vi "processing_steps.vi"(1 "input cluster":T3) -> (0 "output cluster":T1)   [LabVIEW 2010]
uses:
  <vilib>/vision/Image Controls.llb/IMAQ Image.ctl
  lib/MWT.dll
  <vilib>/vision/NI_Vision_Development_Module.lvlib
panel:
  out "Image Pixels (I16) 3":i16[][](array[numeric])
  out "Image Pixels (I16) 2":i16[][](array[numeric])
  out "element 2":i32
  out "element":i32
  out "return type":i32
  out "error out":errorcluster
  out "Numeric":i32
  out "Image Out":T2
  out "Image Pixels (I16)":i16[][](array[numeric])
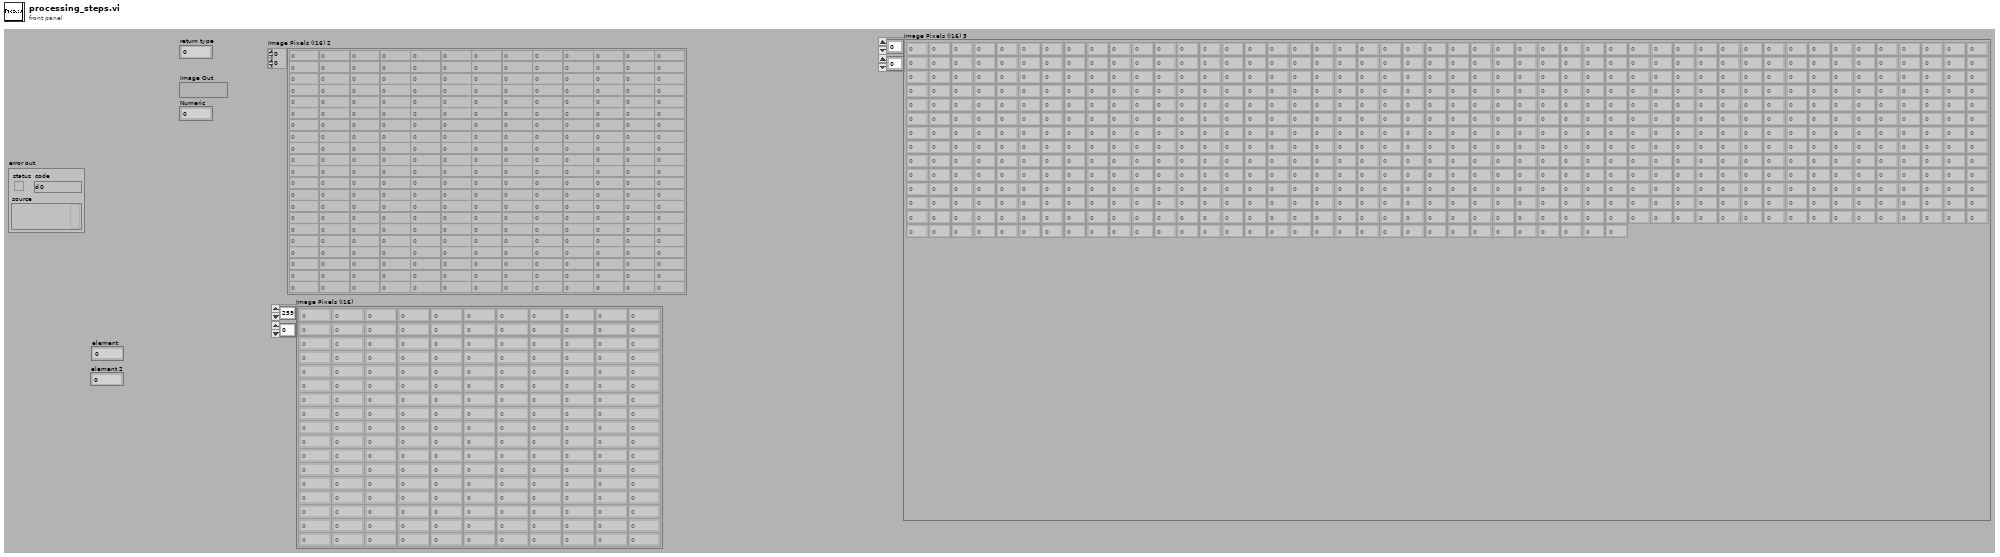
[diagram p1: front panel]
types:
  T1 = cluster{"return value":i32, "return value":i32, "Image Pixels (I16) out":i16[][], "coordinates":i32[]}
  T2 = typedef "IMAQ Image.ctl" = refnum<image>
  T3 = cluster{i32, "Value":i32, "Value":u16, sgl, "Value":u16, "Value":bool, "Value":u32, "Image Out":T2, "Image Pixels (I16)":i16[][], i32[]}
  T4 = typedef "Image Type" = u32
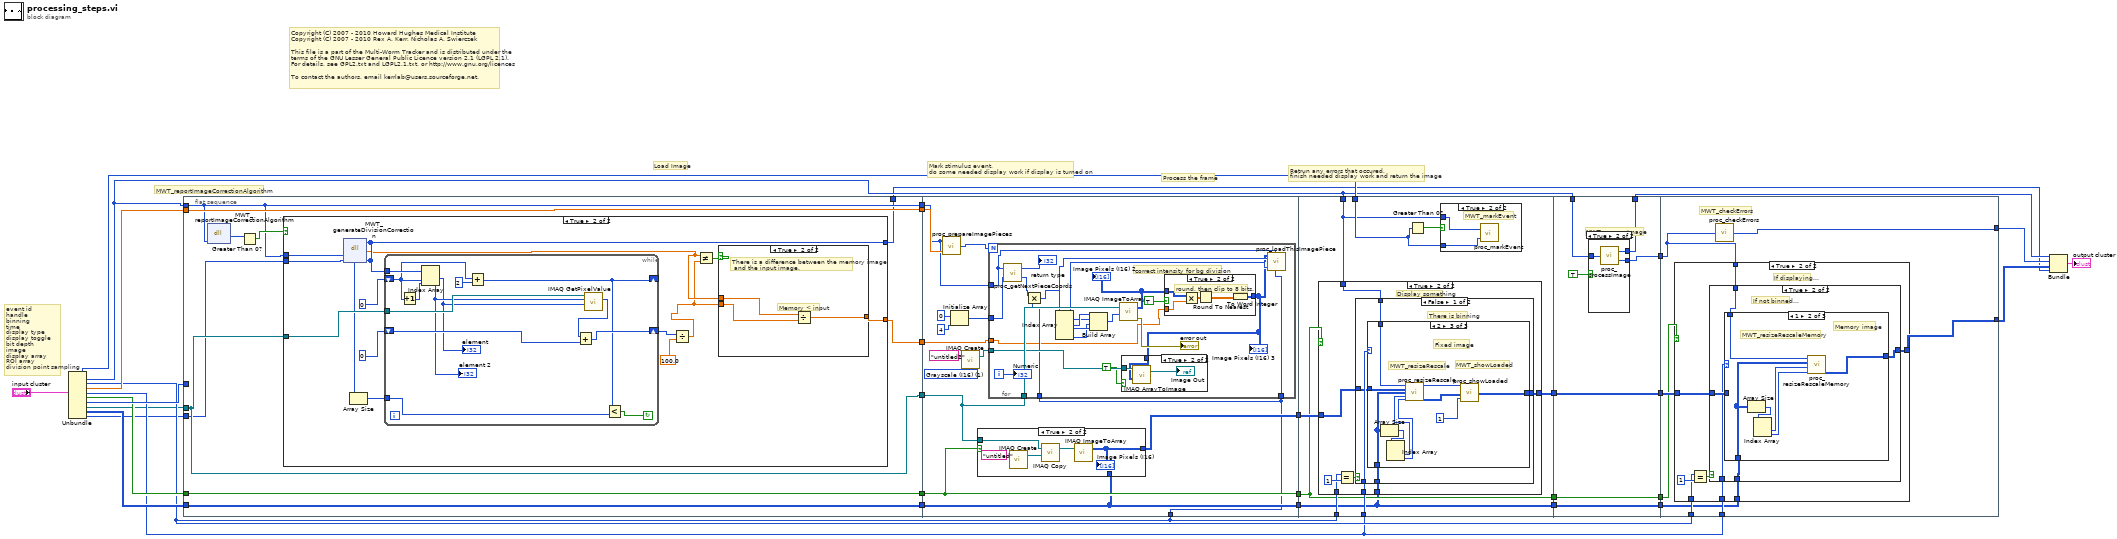
[diagram p0: block diagram]
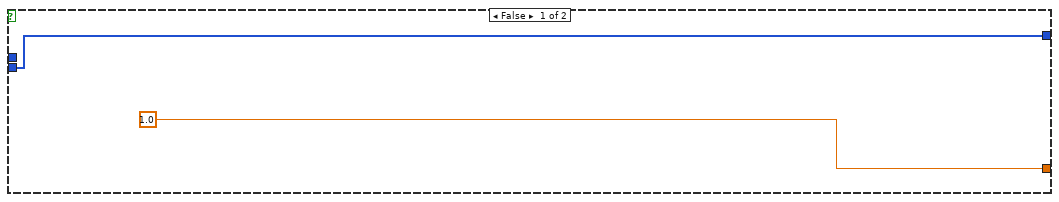
[diagram p2: hidden frame]
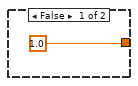
[diagram p3: hidden frame]
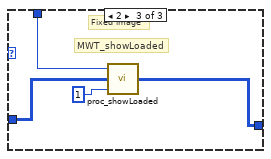
[diagram p12: hidden frame]
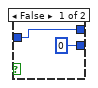
[diagram p14: hidden frame]
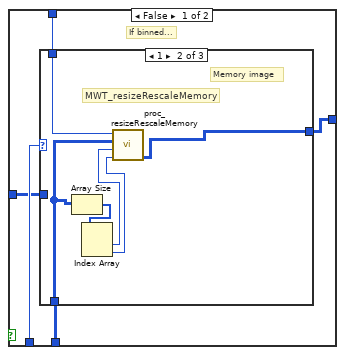
[diagram p16: hidden frame]
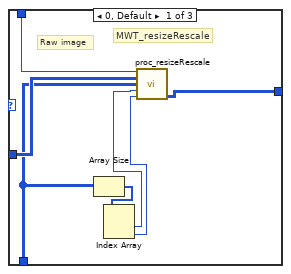
[diagram p17: hidden frame]
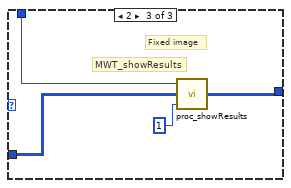
[diagram p18: hidden frame]
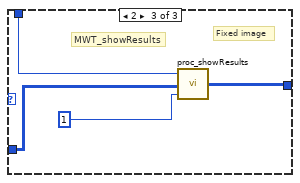
[diagram p20: hidden frame]
diagram:
  # "MWT_reportImageCorrectionAlgorithm"
  # "Copyright (C) 2007 - 2010 Howard Hughes Medical Institute\nCopyright (C) 2007 - 2010 Rex A. Kerr, Nicholas A. Swierczek\n \nThis file is a part of the Multi-Worm Tracker and is distributed under the\nterms of the GNU Lesser General Public Licence version 2.1 (LGPL 2.1).\nFor details, see GPL2.txt and LGPL2.1.txt, or http://www.gnu.org/licences\n \nTo contact the authors, email kerrlab@users.sourceforge.net."
  # "Retrun any errors that occured,\nfinish needed display work and return the image"
  # "Process the frame"
  # "Mark stimulus event,\ndo some needed display work if display is turned on"
  # "Load Image"
  # "event id\nhandle\nbinning\ntime\ndisplay type\ndisplay toggle\nbit depth\nimage\ndisplay array\nROI array\ndivision point sampling"
  n1 = Unbundle("input cluster") -> (w30:i32, "Value"=w5:i32, "Value"=w24:u16, w31:sgl, "Value"=w23:u16, "Value"=w26:bool, "Value"=w32:u32, "Image Out"=w12:T2, "Image Pixels (I16)"=w25:i16[][], w3:i32[])
  n2 = flat-sequence {
    tunnel: w25 -> [w40]
    tunnel: w26 -> [w41]
    tunnel: w5 -> [w36]
    tunnel: w32 -> [_]
    tunnel: w12 -> [w39]
    tunnel: w31 -> [w42]
    tunnel: [w42] -> w11
    tunnel: [w39] -> w10
    tunnel: [w36] -> w9
    tunnel: [w41] -> w8
    tunnel: [w40] -> w7
    tunnel: [w35] -> w6
    tunnel: w3 -> [w34]
    tunnel: [w33] -> w2
    tunnel: [w88] -> w22
    tunnel: [w89] -> w21
    tunnel: [w87] -> w20
    tunnel: w24 -> [w76]
    tunnel: w11 -> [w79]
    tunnel: w10 -> [w83]
    tunnel: w9 -> [w77]
    tunnel: w8 -> [w89]
    tunnel: w7 -> [w87]
    tunnel: w6 -> [w75]
    tunnel: w30 -> [w133]
    tunnel: w24 -> [w132]
    tunnel: w5 -> [w131]
    tunnel: w23 -> [w130]
    tunnel: [w129] -> w19
    tunnel: w22 -> [w128]
    tunnel: w21 -> [w127]
    tunnel: [w127] -> w18
    tunnel: w20 -> [w126]
    tunnel: [w126] -> w17
    tunnel: [w179] -> w16
    tunnel: [w180] -> w27
    tunnel: w5 -> [w178]
    tunnel: [w177] -> w15
    tunnel: w19 -> [w177]
    tunnel: [w176] -> w14
    tunnel: w18 -> [w176]
    tunnel: [w175] -> w13
    tunnel: w17 -> [w175]
    tunnel: w16 -> [w191]
    tunnel: [w190] -> w28
    tunnel: [w193] -> w29
    tunnel: w24 -> [w192]
    tunnel: w23 -> [w189]
    tunnel: w15 -> [w188]
    tunnel: w14 -> [w187]
    tunnel: w13 -> [w186]
    frame #0 {
      n3 = dll-call lib="C:/MWT/lib/MWT.dll" fn="MWT_reportImageCorrectionAlgorithm"("handle"=w36) -> ("return type"=w38:i32)  [unwired: 4 in, 2 out]
      n4 = Greater Than 0?(x=w38) -> (x > 0?=w37:bool)
      n5 = case shown="True" w37 {
        tunnel: w36 -> [_ w57]
        tunnel: w39 -> [_ w54]
        tunnel: [1.0 w52] -> w35
        tunnel: w34 -> [w43 w49]
        tunnel: [w43 w48] -> w33
        frame False {
        }
        frame True {
          n6 = dll-call lib="C:/MWT/lib/MWT.dll" fn="MWT_generateDivisionCorrection"("handle"=w57, "coordinates"=w49) -> ("return type"=w47:sgl, "coordinates"=w48:i32[])  [unwired: 4 in, 2 out]
          n7 = Array Size(array=w48) -> (size(s)=w45:i32)
          n8 = while {
            shift-right: [w59] -> _
            shift-left: 0 -> [w67]
            tunnel: w48 -> [w69]
            tunnel: w54 -> [w66]
            shift-right: [w63] -> w50
            shift-left: i16 0 -> [w64]
            tunnel: w45 -> [w58]
            stop <- w60 continue-if-true
            n9 = Increment(x=w67) -> (x+1=w70:i32)
            n10 = Index Array(array=w69, index #1=w67, index #2=w70) -> (element #1=w61:i32, element #2=w62:i32)
            "element" <- w61
            "element 2" <- w62
            n11 = Add(x=w67, y=2) -> (x+y=w59:i32)
            n12 = call "IMAQ GetPixelValue"("Image"=w66, "X Coordinate"=w62, "Y Coordinate"=w61) -> ("Pixel Value (I16)"=w65:i16)  [unwired: 3 in, 4 out]
            n13 = Add(x=w65, y=w64) -> (x+y=w63:i16)
            n14 = Less?(x=w59, y=w58) -> (x < y?=w60:bool)
          }
          n15 = Divide(x=w50, y=sgl 100.0) -> (x/y=w46:sgl)
          n16 = Not Equal?(x=w47, y=w46) -> (x != y?=w53:bool)
          n17 = case shown="True" w53 {
            tunnel: w47 -> [_ w74]
            tunnel: w46 -> [_ w73]
            tunnel: [1.0 w72] -> w52
            frame False {
            }
            frame True {
              # "Memory < input"
              # "There is a difference between the memory image\n and the input image."
              n18 = Divide(x=w74, y=w73) -> (x/y=w72:sgl)
            }
          }
        }
      }
    }
    frame #1 {
      w80 = T4 1 items=["Grayscale (U8)", "Grayscale (I16)", "Grayscale (SGL)", "Complex (CSG)", "RGB (U32)", "HSL (U32)", "RGB (U64)"] ("Image Type")
      n19 = call "proc_prepareImagePieces.vi"("time"=w79, "handle"=w77) -> ("piece count"=w78:i32)
      n20 = Initialize Array(0 ("element"), 4 ("dimension size")) -> (w84:i32[])
      n21 = call "IMAQ Create"("Image Name"="untitled2", "Image Type"=w80) -> ("New Image"=w81:T2)  [unwired: 3 in, 1 out]
      n22 = case shown="True" w89 {
        tunnel: [w120 w125] -> w88
        tunnel: w87 -> [w120 _]
        tunnel: w83 -> [_ w121]
        frame False {
        }
        frame True {
          n23 = call "IMAQ Create"("Image Name"="untitled") -> ("New Image"=w123:T2)  [unwired: 4 in, 1 out]
          n24 = call "IMAQ Copy"("Image Dst"=w123, "Image Src"=w121) -> ("Image Dst Out"=w122:T2)  [unwired: 4 in, 1 out]
          n25 = call "IMAQ ImageToArray"("Image"=w122) -> ("Image Pixels (I16)"=w125:i16[][])  [unwired: 3 in, 4 out]
          "Image Pixels (I16)" <- w125
        }
      }
      n26 = for {
        N: w78 -> [_]
        tunnel: w77 -> [w104]
        tunnel: w84 -> [w106]
        tunnel: w83 -> [w110]
        tunnel: w81 -> [w109]
        tunnel: w76 -> [w97]
        tunnel: w76 -> [w96]
        tunnel: w75 -> [w90]
        i -> [w108]
        # "correct intensity for bg division"
        n27 = call "proc_getNextPieceCoords.vi"("initialized array"=w106, "handle"=w104) -> ("coordinates"=w95:i32[], "returned handle"=→"return type":i32)
        n28 = Multiply(x=w95, y=w96) -> (x*y=w94:i32[])
        n29 = Index Array(array=w94) -> (element #1=w99:i32, element #2=w100:i32, element #3=w103:i32, element #4=w102:i32)  [unwired: 4 in]
        n30 = Build Array(w100, w99, w102, w103) -> (w98:i32[])
        n31 = call "IMAQ ImageToArray"("Optional Rectangle"=w98, "Image"=w110) -> ("error out"=→"error out":errorcluster, "Image Pixels (I16)"=w92:i16[][])  [unwired: 2 in, 3 out]
        "Image Pixels (I16) 2" <- w92
        n32 = case shown="True" TRUE {
          tunnel: w90 -> [_ w116]
          tunnel: [w111 w113] -> w93
          tunnel: w92 -> [w111 w115]
          frame False {
          }
          frame True {
            # "round, then clip to 8 bits."
            n33 = Multiply(x=w115, y=w116) -> (x*y=w114:dbl[][])
            n34 = Round To Nearest(number=w114) -> (nearest integer value=w112:dbl[][])
            n35 = To Word Integer(number=w112) -> (16bit integer=w113:i16[][])
          }
        }
        "Image Pixels (I16) 3" <- w93
        n36 = case shown="True" TRUE {
          tunnel: w109 -> [_ w119]
          tunnel: w93 -> [_ w117]
          frame False {
          }
          frame True {
            n37 = call "IMAQ ArrayToImage"("Image Pixels (I16)"=w117, "Image"=w119) -> ("Image Out"=→"Image Out":T2)  [unwired: 8 in, 1 out]
          }
        }
        n38 = call "proc_loadThisImagePiece.vi"("Image Pixels (I16)"=w93, "handle"=w104, "x"=w99, "y"=w100, "bin value"=w97) -> ()  [unwired: 1 in, 1 out]
        "Numeric" <- w108
      }
    }
    frame #2 {
      n39 = case shown="True" w127 {
        tunnel: [w135 w143] -> w129
        tunnel: w132 -> [_ w140]
        tunnel: w131 -> [_ w139]
        tunnel: w130 -> [_ w138]
        tunnel: w126 -> [_ w137]
        tunnel: w128 -> [w135 w136]
        frame False {
          # "Display nothing"
        }
        frame True {
          # "Display something"
          n40 = Equal?(x=w140, y=1) -> (x = y?=w142:bool)
          n41 = case shown="False" w142 {
            tunnel: [w148 w165] -> w143
            tunnel: w139 -> [w147 w163]
            tunnel: w138 -> [w146 w161]
            tunnel: w137 -> [w145 w164]
            tunnel: w136 -> [w144 w162]
            frame False {
              # "There is binning"
              n42 = case shown="2" w146 {
                tunnel: [w149 w150 w160] -> w148
                tunnel: w147 -> [_ _ w156]
                tunnel: w145 -> [_ _ w154]
                tunnel: w144 -> [w149 w150 w155]
                frame 0, Default {
                  # "Raw image"
                }
                frame 1 {
                  # "Memory image"
                }
                frame 2 {
                  # "MWT_showLoaded"
                  # "MWT_resizeRescale"
                  # "Fixed image"
                  n43 = Array Size(array=w154) -> (size(s)=w153:i32[])
                  n44 = Index Array(array=w153) -> (element #1=w152:i32, element #2=w151:i32)  [unwired: 2 in]
                  n45 = call "proc_resizeRescale.vi"("handle"=w156, "Source Image Pixels (I16)"=w155, "Destination Image Pixels (I16)"=w154, "to_width"=w152, "to_height"=w151) -> ("handle out"=w158:i32, "Image Pixels (I16) out"=w157:i16[][])  [unwired: 9 in]
                  n46 = call "proc_showLoaded.vi"("bin value"=1 ("bin"), "Image Pixels (I16)"=w157, "handle"=w158) -> ("Image Pixels (I16) out"=w160:i16[][])
                }
              }
            }
            frame True {
              # "There is no binning"
              n47 = case shown="1" w161 {
                tunnel: [w166 w167 w171] -> w165
                tunnel: w164 -> [_ _ _]
                tunnel: w163 -> [_ _ w169]
                tunnel: w162 -> [w166 w167 w168]
                frame 0, Default {
                  # "Raw image"
                }
                frame 1 {
                  # "Memory image"
                }
                frame 2 {
                  # "MWT_showLoaded"
                  # "Fixed image"
                  n48 = call "proc_showLoaded.vi"("bin value"=1 ("bin"), "Image Pixels (I16)"=w168, "handle"=w169) -> ("Image Pixels (I16) out"=w171:i16[][])
                }
              }
            }
          }
        }
      }
      n49 = Greater Than 0?(x=w133) -> (x > 0?=w134:bool)
      n50 = case shown="True" w134 {
        tunnel: w133 -> [_ w173]
        tunnel: w131 -> [_ w172]
        frame False {
        }
        frame True {
          # "MWT_markEvent"
          n51 = call "proc_markEvent.vi"("event_type"=w173, "handle"=w172) -> ()
        }
      }
    }
    frame #3 {
      # "MWT_processImage"
      n52 = case shown="True" TRUE {
        tunnel: [w182 w185] -> w180
        tunnel: [0 ("output handle") w184] -> w179
        tunnel: w178 -> [w182 w183]
        frame False {
        }
        frame True {
          n53 = call "proc_processImage.vi"("handle"=w183) -> ("return value"=w185:i32, "handle out"=w184:i32)
        }
      }
    }
    frame #4 {
      # "MWT_checkErrors"
      n54 = case shown="True" w187 {
        tunnel: w191 -> [_ w202]
        tunnel: [w194 w201] -> w193
        tunnel: w186 -> [_ w200]
        tunnel: w192 -> [_ w197]
        tunnel: w189 -> [_ w196]
        tunnel: w188 -> [w194 w195]
        frame False {
        }
        frame True {
          # "If displaying..."
          n55 = Equal?(x=w197, y=1) -> (x = y?=w199:bool)
          n56 = case shown="True" w199 {
            tunnel: w202 -> [w207 w227]
            tunnel: [w206 w229] -> w201
            tunnel: w200 -> [w205 w228]
            tunnel: w196 -> [w204 w225]
            tunnel: w195 -> [w203 w226]
            frame False {
              # "If binned..."
              n57 = case shown="1" w204 {
                tunnel: w207 -> [w214 w220 w223]
                tunnel: [w213 w215 w221] -> w206
                tunnel: w205 -> [w210 w219 _]
                tunnel: w203 -> [w212 _ w222]
                frame 0, Default {
                  # "MWT_resizeRescale"
                  # "Raw image"
                  n58 = Array Size(array=w210) -> (size(s)=w211:i32[])
                  n59 = Index Array(array=w211) -> (element #1=w209:i32, element #2=w208:i32)  [unwired: 2 in]
                  n60 = call "proc_resizeRescale.vi"("handle"=w214, "Source Image Pixels (I16)"=w212, "Destination Image Pixels (I16)"=w210, "to_width"=w209, "to_height"=w208) -> ("Image Pixels (I16) out"=w213:i16[][])  [unwired: 9 in, 1 out]
                }
                frame 1 {
                  # "MWT_resizeRescaleMemory"
                  # "Memory image"
                  n61 = Array Size(array=w219) -> (size(s)=w218:i32[])
                  n62 = Index Array(array=w218) -> (element #1=w217:i32, element #2=w216:i32)  [unwired: 2 in]
                  n63 = call "proc_resizeRescaleMemory.vi"("to_height"=w216, "to_width"=w217, "Image Pixels (I16)"=w219, "handle"=w220) -> ("Image Pixels (I16) out"=w215:i16[][])  [unwired: 6 in, 1 out]
                }
                frame 2 {
                  # "MWT_showResults"
                  # "Fixed image"
                  n64 = call "proc_showResults.vi"("bin value"=1 ("bin"), "Image Pixels (I16)"=w222, "handle"=w223) -> ("Image Pixels (I16) out"=w221:i16[][])
                }
              }
            }
            frame True {
              # "If not binned..."
              n65 = case shown="1" w225 {
                tunnel: w227 -> [_ w236 w239]
                tunnel: [w230 w235 w238] -> w229
                tunnel: w228 -> [_ w231 _]
                tunnel: w226 -> [w230 _ w237]
                frame 0, Default {
                  # "Raw image"
                }
                frame 1 {
                  # "MWT_resizeRescaleMemory"
                  # "Memory image"
                  n66 = Array Size(array=w231) -> (size(s)=w234:i32[])
                  n67 = Index Array(array=w234) -> (element #1=w232:i32, element #2=w233:i32)  [unwired: 2 in]
                  n68 = call "proc_resizeRescaleMemory.vi"("to_height"=w233, "to_width"=w232, "Image Pixels (I16)"=w231, "handle"=w236) -> ("Image Pixels (I16) out"=w235:i16[][])  [unwired: 6 in, 1 out]
                }
                frame 2 {
                  # "MWT_showResults"
                  # "Fixed image"
                  n69 = call "proc_showResults.vi"("bin value"=1 ("bin"), "Image Pixels (I16)"=w237, "handle"=w239) -> ("Image Pixels (I16) out"=w238:i16[][])
                }
              }
            }
          }
        }
      }
      n70 = call "proc_checkErrors.vi"("handle"=w191) -> ("return value"=w190:i32)
    }
  }
  n71 = Bundle("return value"=w27, "return value"=w28, "Image Pixels (I16) out"=w29, "coordinates"=w2) -> (→"output cluster":T1)  [unwired: 1 in]
